vi "ELVIS III v1.0 Build MUX Configuration I2C.vi"(11 "Channel":T4) -> (1 "Configuration Bitmask Array":bool[][](array[boolean]), 2 "Configuration BitCode Array":bool[][](array[boolean]), 3 "Channel Reservation List":T1)   [LabVIEW 2021]
uses:
  <vilib>/myRIO/Common/Instrument Driver Framework/myRIO v1.0/I2C/typedefs/I2C Channels Enum.ctl
  <vilib>/myRIO/Common/Instrument Driver Framework/ELVIS III v1.0/Resource Manager/typedefs/ELVIS III v1.0 Channel Reservation List.ctl
  <vilib>/myRIO/Common/Instrument Driver Framework/ELVIS III v1.0/Resource Manager/typedefs/ELVIS III v1.0 Channel Reservation Info.ctl
  <vilib>/myRIO/Common/Instrument Driver Framework/ELVIS III v1.0/Resource Manager/typedefs/ELVIS III v1.0 Connector List.ctl
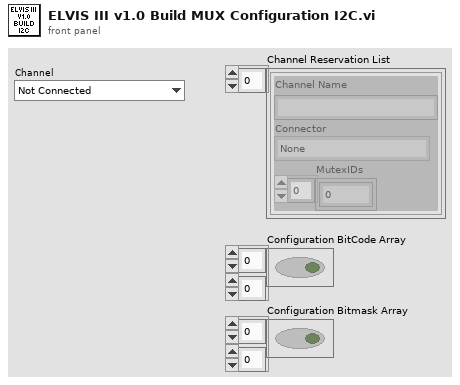
[diagram p1: front panel]
types:
  T1 = typedef "ELVIS III v1.0 Channel Reservation List.ctl" = T2[]
  T2 = typedef "ELVIS III v1.0 Channel Reservation Info.ctl" = cluster{"Channel Name":string, "Connector":T3, "MutexIDs":u32[]}
  T3 = typedef "ELVIS III v1.0 Connector List.ctl" = enum32{"None", "ConnectorA", "ConnectorB"}
  T4 = typedef "I2C Channels Enum.ctl" = enum16{"Not Connected", "A/I2C", "B/I2C", "I2C/I2C"}
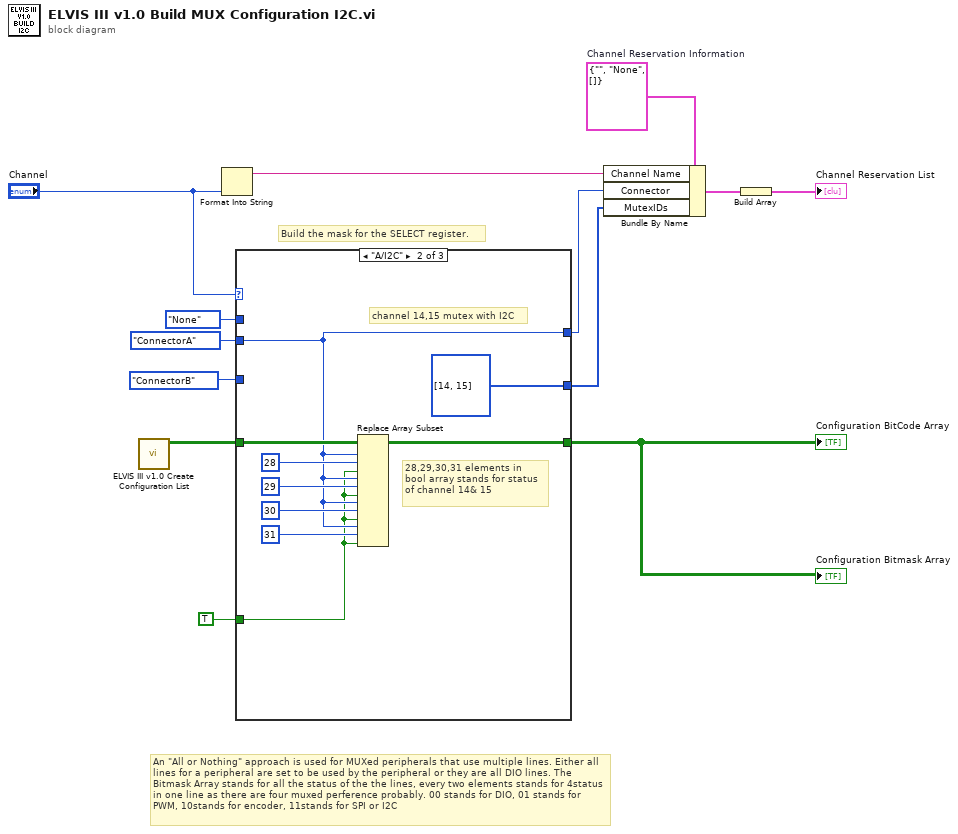
[diagram p0: block diagram]
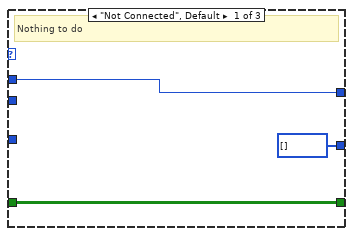
[diagram p2: hidden frame]
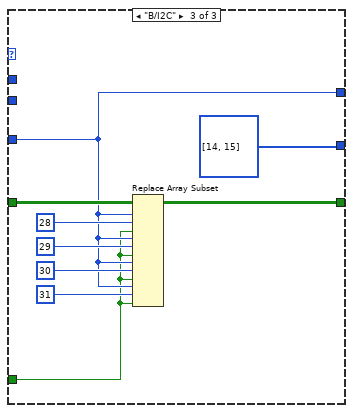
[diagram p3: hidden frame]
diagram:
  w5 = T2 {"Channel Name"="", "Connector"=enum."None", "MutexIDs"=[]}  # Channel Reservation Information
  # "An \"All or Nothing\" approach is used for MUXed peripherals that use multiple lines. Either all lines for a peripheral are set to be used by the peripheral or they are all DIO lines. The Bitmask Array stands for all the status of the the lines, every two elements stands for 4status in one line as there are four muxed perference probably. 00 stands for DIO, 01 stands for PWM, 10stands for encoder, 11stands for SPI or I2C"
  # "Build the mask for the SELECT register."
  n1 = call <vilib>:"ELVIS III v1.0 Create Configuration List.vi"() -> ("Bitmask Array"=w6:bool[][])  [unwired: 11 in]
  n2 = Format Into String("Channel") -> (resulting string=w10:string)  [unwired: 3 in, 1 out]
  n3 = case shown="\"A/I2C\"" "Channel" {
    tunnel: w6 -> [w16 w25 w30]
    tunnel: [w16 w19 w28] -> w1
    tunnel: ELVIS_III_v1.0_Connector_List."None" ("Connector List") -> [w15 _ _]
    tunnel: ELVIS_III_v1.0_Connector_List."ConnectorA" ("Connector List") -> [_ w20 _]
    tunnel: TRUE ("new element/subarray") -> [_ w18 w27]
    tunnel: [w15 w20 w29] -> w7
    tunnel: ELVIS_III_v1.0_Connector_List."ConnectorB" ("Connector List") -> [_ _ w29]
    tunnel: [u32[] [] u32[] [14, 15] u32[] [14, 15]] -> w2
    frame "Not Connected", Default {
      # "Nothing to do"
    }
    frame "A/I2C" {
      # "28,29,30,31 elements in\nbool array stands for status\nof channel 14& 15"
      # "channel 14,15 mutex with I2C"
      n4 = Replace Array Subset(array=w25, new element #1=w18, index (row) #1=w20, index (col) #1=28 ("disabled index (col)"), new element #2=w18, index (row) #2=w20, index (col) #2=29 ("disabled index (col)"), new element #3=w18, index (row) #3=w20, index (col) #3=30 ("disabled index (col)"), new element #4=w18, index (row) #4=w20, index (col) #4=31 ("disabled index (col)")) -> (w19:bool[][])
    }
    frame "B/I2C" {
      n5 = Replace Array Subset(array=w30, new element #1=w27, index (row) #1=w29, index (col) #1=28 ("disabled index (col)"), new element #2=w27, index (row) #2=w29, index (col) #2=29 ("disabled index (col)"), new element #3=w27, index (row) #3=w29, index (col) #3=30 ("disabled index (col)"), new element #4=w27, index (row) #4=w29, index (col) #4=31 ("disabled index (col)")) -> (w28:bool[][])
    }
  }
  "Configuration BitCode Array" <- w1
  "Configuration Bitmask Array" <- w1
  n6 = Bundle By Name(cluster=w5, "Channel Name"=w10, "Connector"=w7, "MutexIDs"=w2) -> (w9:T2)
  n7 = Build Array(w9) -> (→"Channel Reservation List":T2[])
